vi "Define Server Stats.vi"(9 "Port locations":string[](array[string]), 10 "scan rate (Hz)":dbl, 11 "Refnum in":refnum<k21>) -> (1 "Channels":refnum<k21>[](array[refnum]), 2 "NumChans":u32, 3 "Server Stats":T1={"scan rate"=10.0, "# connections"=0, "channel settings"=[]} {"channel settings"."lower input limits" format="%.4f"; "channel settings"."upper input limits" format="%.4f"; "scan rate" format="%.2f"})   [LabVIEW 2015]
uses:
  <resource>/objmgr/daqmx.rc
  DataServer/Server stats.ctl
panel:
  # "Hz"
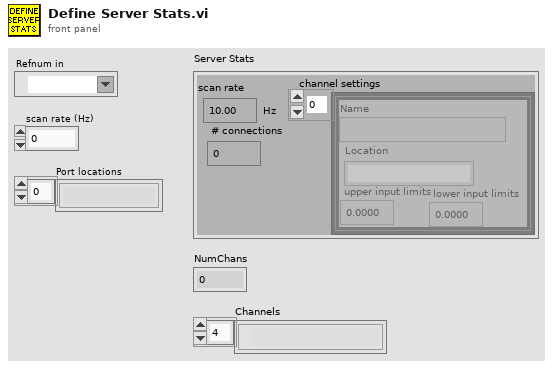
[diagram p1: front panel]
types:
  T1 = typedef "Server stats.ctl" = cluster{"scan rate":dbl, "# connections":i32, "channel settings":cluster{"Name":string, "upper input limits":sgl, "lower input limits":sgl, "Location":string}[]}
  T2 = cluster{"Name":string, "upper input limits":sgl, "lower input limits":sgl, "Location":string}[]
  T3 = cluster{"Name":string, "upper input limits":sgl, "lower input limits":sgl, "Location":string}
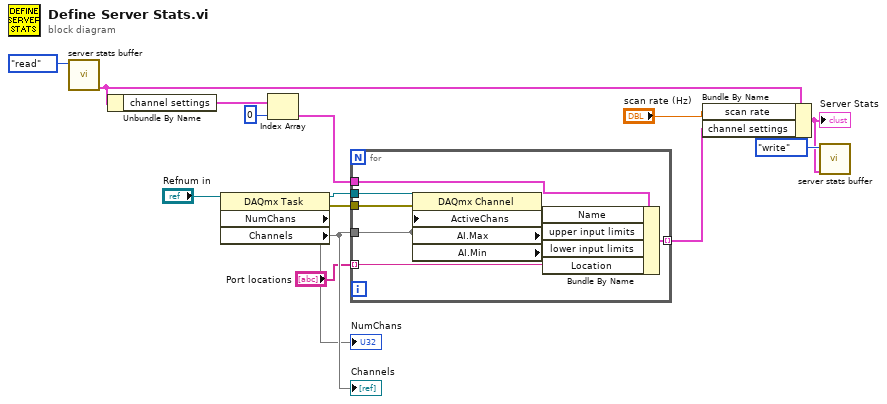
[diagram p0: block diagram]
diagram:
  n1 = call "server stats buffer.vi"("state"=enum16{"write", "read", "change connections"}."read") -> ("Server Stats out"=w5:T1)  [unwired: 6 in]
  n2 = Unbundle By Name(w5) -> ("channel settings"=w6:T2)
  n3 = property class="DAQmx Task"(reference="Refnum in") -> (reference out=w13:refnum<k21>, error out=w12:errorcluster, "NumChans"=→"NumChans", "Channels"=w15)  [unwired: 1 in]
  "Channels" <- w15
  n4 = Index Array(array=w6, index=0) -> (element=w8:T3)
  n5 = for {
    tunnel: w12 -> [w23]
    tunnel: w13 -> [w22]
    tunnel: w8 -> [w21]
    tunnel: "Port locations" -> [w20] mode=indexing
    tunnel: [w19] -> w10 mode=indexing
    tunnel: w15 -> [w18]
    n6 = property class="DAQmx Channel"(reference=w22, error in=w23, "ActiveChans"=w18) -> ("AI.Max"=w16, "AI.Min"=w17)  [unwired: 2 out]
    n7 = Bundle By Name(cluster=w21, "Name"=w18, "upper input limits"=w16, "lower input limits"=w17, "Location"=w20) -> (w19:T3)
  }
  n8 = Bundle By Name(cluster=w5, "scan rate"="scan rate (Hz)", "channel settings"=w10) -> (w1:T1)
  "Server Stats" <- w1
  n9 = call "server stats buffer.vi"("Server Stats in"=w1, "state"=enum16{"write", "read", "change connections"}."write") -> ()  [unwired: 5 in, 1 out]
